vi "test_Add Single Ch. Enumerated List .vi"(8 "error in (no error)":errorcluster, 11 "TestCase in":refnum<class "Instrument Addon Scripting API Channels Unit Tests.lvclass">) -> (0 "error out":errorcluster, 3 "TestCase out":refnum<class "Instrument Addon Scripting API Channels Unit Tests.lvclass">)   [LabVIEW 2018, in "Instrument Addon Scripting API Channels Unit Tests.lvclass"]
uses:
  Instrument Addon Scripting API Channels Unit Tests.lvclass
  APIs/Scripting API/TypeDefs/Single Channel Enumerated List Settings.ctl
  Instrument Addon Scripting API Channels Unit Tests.lvclass/Instrument Addon Scripting API Channels Unit Tests.ctl
  Addon/Addon Shared/SubVIs/Constants.vi
  <vilib>/NI/NI VeriStand Advanced SysDef API/_SubVIs/SysDef.Search.GUID.vi
  <vilib>/NI/NI VeriStand Advanced SysDef API/_SubVIs/SysDef.Search.GUIDs.vi
  APIs/Scripting API/Channels/Create Data Channel - Single Channel - Enumerated List.vi
  <vilib>/NI Veristand/Custom Device API/Get Item Property (String Array).vi
  <vilib>/addons/_JKI Toolkits/VI Tester/TestCase.llb/TestCase.lvclass
  Instrument Addon Scripting API Test Assets/Instrument Addon Scripting API Test Assets.lvclass
  <vilib>/NI/NI VeriStand Advanced SysDef API/SysDef API/Advanced System Definition.lvlib
  Addon/Addon Shared/Instrument Addon Shared.lvlib
  APIs/Scripting API/Instrument Addon Scripting API.lvlib
  <vilib>/NI Veristand/Custom Device API/Custom Device API.lvlib
  C:/Program Files (x86)/National Instruments/LabVIEW 2018/vi.lib/addons/_JKI Toolkits/VI Tester/TestCase.llb/TestCase.lvclass
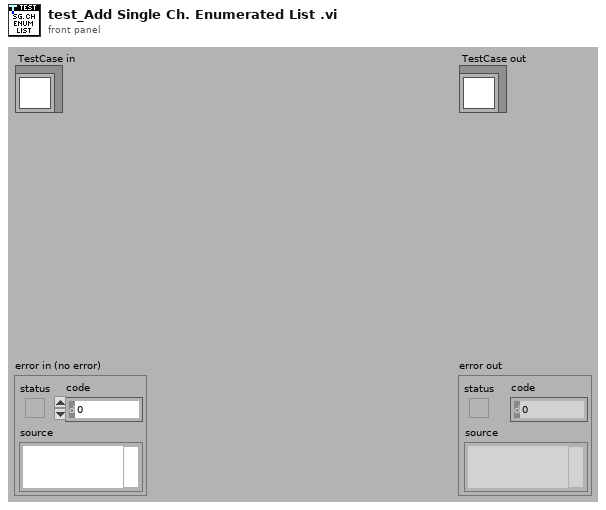
[diagram p1: front panel]
types:
  T1 = typedef "Instrument Addon Scripting API.lvlib/Single Channel Enumerated List Settings.ctl" = cluster{"Enumerated List":string[], "Default Value":dbl, "Units":string}
  T2 = typedef "Custom Device API.lvlib/Custom Device Item Ref.ctl" = u64
  T3 = typedef "Custom Device API.lvlib/Custom Device Channel.ctl" = cluster{"Type":T4, "Units":string, "Default Value":dbl, "Faultable":bool, "Scalable":bool}
  T4 = typedef "Custom Device API.lvlib/Custom Device Channel Type.ctl" = enum16{"Input", "Output"}
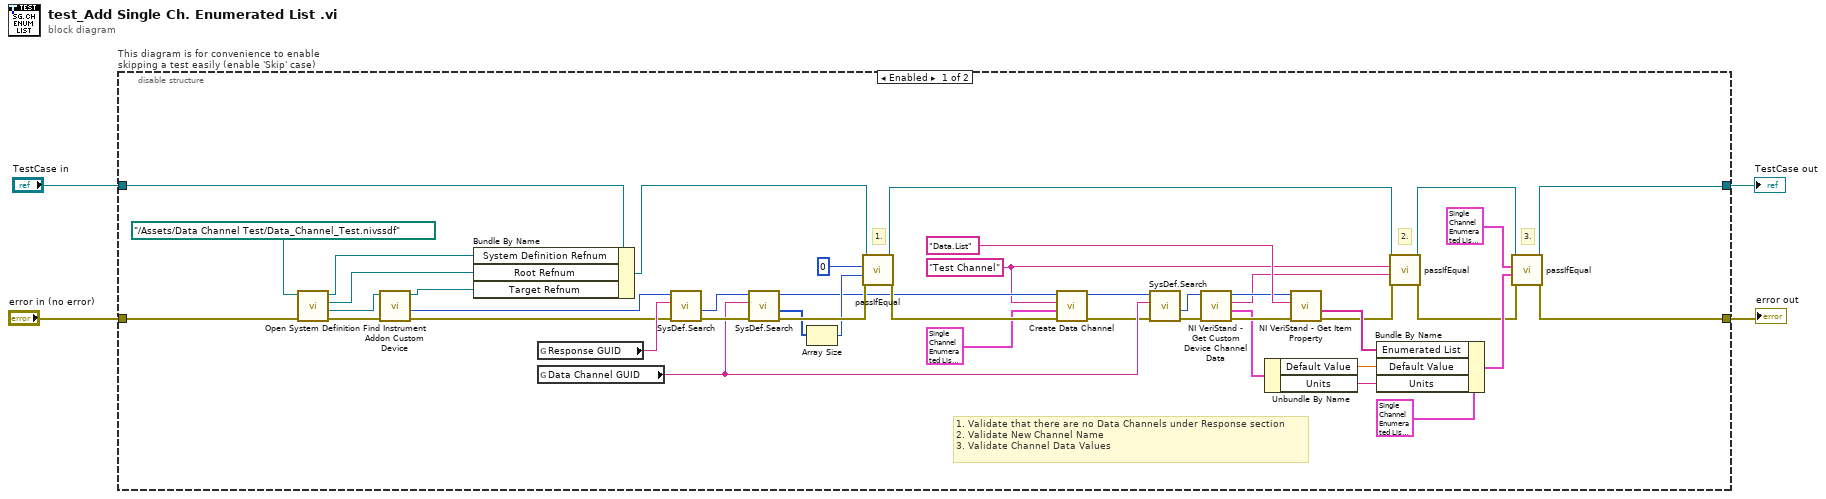
[diagram p0: block diagram]
diagram:
  n1 = disable-structure "This diagram is for convenience to enable skipping a test easily (enable 'Skip' case)" shown="Enabled" {
    disable-tunnel: "TestCase in" -> [w6 w52]
    disable-tunnel: [w48 w50] -> w1
    disable-tunnel: [w47 w51] -> w3
    disable-tunnel: "error in (no error)" -> [w43 w49]
    frame Enabled {
      w14 = "Test Channel" ("Name")
      # "3."
      # "2."
      # "1. Validate that there are no Data Channels under Response section\n2. Validate New Channel Name\n3. Validate Channel Data Values"
      # "1."
      n2 = call "Open System Definition.vi"("error in (no error)"=w43, "System Definition File"=path "../Assets/Data Channel Test/Data_Channel_Test.nivssdf") -> ("error out"=w46:errorcluster, "Target Refnum"=w45:refnum<k24>, "Root Refnum"=w9:refnum<k24>, "System Definition Refnum"=w10:refnum<k24>)  [unwired: 6 in]
      n3 = call "Find Instrument Addon Custom Device.vi"("error in"=w46, "target in"=w45) -> ("error out"=w7:errorcluster, "NodeID"=w42:u64, "target out"=w8:refnum<k24>)  [unwired: 7 in]
      n4 = Bundle By Name(cluster=w6, "System Definition Refnum"=w10, "Root Refnum"=w9, "Target Refnum"=w8) -> (w5:refnum<class "Instrument Addon Scripting API Channels Unit Tests.lvclass">)
      n5 = global read "Constants.vi" "Response GUID"() -> (w41:string)
      n6 = global read "Constants.vi" "Data Channel GUID"() -> (w38:string)
      n7 = call-poly <vilib>:"SysDef.Search.vi"("error in (no error)"=w7, "GUID"=w41, "nodeID"=w42) -> ("error out"=w39:errorcluster, "Value out"=w40:u64)  [unwired: 5 in, 2 out]
      n8 = call-poly <vilib>:"SysDef.Search.vi"("error in (no error)"=w39, "GUID"=w38, "nodeID"=w40) -> ("error out"=w21:errorcluster, "Values Out"=w20:u64[], "nodeID out"=w15:u64)  [unwired: 5 in, 1 out]
      n9 = Array Size(array=w20) -> (size(s)=w19:i32)
      n10 = call-dynamic "passIfEqual.vi"("error in (no error)"=w21, "y"=w19, "x"=0 ("size(s)"), "TestCase in"=w5) -> ("error out"=w16:errorcluster, "TestCase out"=w22:refnum<class "Instrument Addon Scripting API Channels Unit Tests.lvclass">)  [unwired: 6 in]
      n11 = call-poly "Create Data Channel.vi"("Error In"=w16, "Settings"=T1 {"Enumerated List"=["Test List Element 1"], "Default Value"=10.0, "Units"="ms"}, "Name"=w14, "Message Refnum In"=w15) -> ("Error Out"=w11:errorcluster, "Message Refnum Out"=w12:T2)  [unwired: 5 in, 1 out]
      n12 = call-poly <vilib>:"SysDef.Search.vi"("error in (no error)"=w11, "GUID"=w38, "nodeID"=w12) -> ("error out"=w37:errorcluster, "Value out"=w36:u64)  [unwired: 5 in, 2 out]
      n13 = call <vilib>:"NI VeriStand - Get Custom Device Channel Data.vi"("error in (no error)"=w37, "Channel Ref in"=w36) -> ("error out"=w35:errorcluster, "Channel"=w32:T3, "Channel Name"=w26:string, "Channel Ref out"=w28:T2)  [unwired: 4 in, 2 out]
      n14 = Unbundle By Name(w32) -> ("Default Value"=w31:dbl, "Units"=w30:string)
      n15 = call-poly <vilib>:"NI VeriStand - Get Item Property.vi"("error in (no error)"=w35, "Property Name"="Data.List", "Item Ref in"=w28) -> ("error out"=w24:errorcluster, "Value"=w33:string[])  [unwired: 5 in, 2 out]
      n16 = Bundle By Name(cluster=T1 {"Enumerated List"=["Test List Element 1"], "Default Value"=10.0, "Units"="ms"} ("Settings"), "Enumerated List"=w33, "Default Value"=w31, "Units"=w30) -> (w25:T1)
      n17 = call-dynamic "passIfEqual.vi"("error in (no error)"=w24, "y"=w26, "x"=w14, "TestCase in"=w22) -> ("error out"=w23:errorcluster, "TestCase out"=w27:refnum<class "Instrument Addon Scripting API Channels Unit Tests.lvclass">)  [unwired: 6 in]
      n18 = call-dynamic "passIfEqual.vi"("error in (no error)"=w23, "y"=w25, "x"=T1 {"Enumerated List"=["Test List Element 1"], "Default Value"=10.0, "Units"="ms"} ("Settings"), "TestCase in"=w27) -> ("error out"=w47:errorcluster, "TestCase out"=w48:refnum<class "Instrument Addon Scripting API Channels Unit Tests.lvclass">)  [unwired: 6 in]
    }
    frame Disabled {
      # "skip test result while test is under development"
      n19 = call <vilib>:"skip.vi"("error in (no error)"=w49, "TestCase in"=w52) -> ("error out"=w51:errorcluster, "TestCase out"=w50:refnum<class "Instrument Addon Scripting API Channels Unit Tests.lvclass">)  [unwired: 8 in]
    }
  }
  "error out" <- w3
  "TestCase out" <- w1
